vi "sub build w data.vi"(8 "error in":errorcluster, 11 "<w> data":T1) -> (0 "error out":errorcluster, 3 "<w> string":string)   [LabVIEW 2018, in "Frame Analizer.lvclass"]
uses:
  Frame Analizer.lvclass
  frame w data.ctl
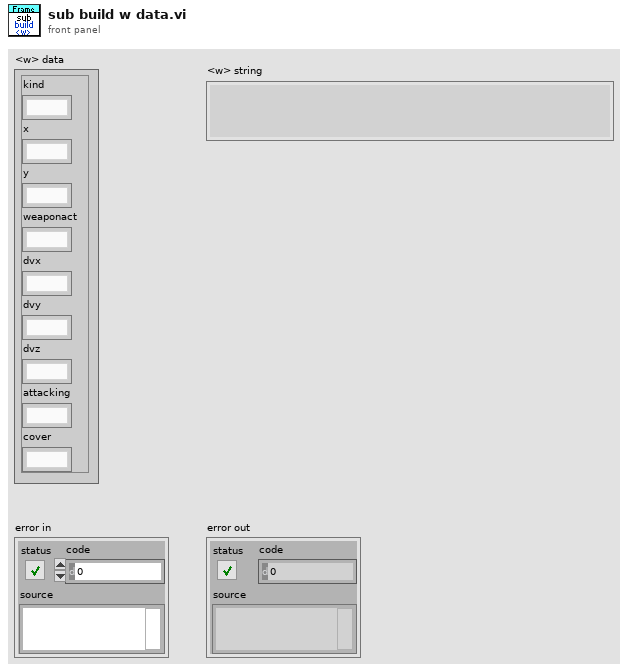
[diagram p1: front panel]
types:
  T1 = typedef "Frame Analizer.lvclass/frame w data.ctl" = cluster{"kind":string, "x":string, "y":string, "weaponact":string, "dvx":string, "dvy":string, "dvz":string, "attacking":string, "cover":string}
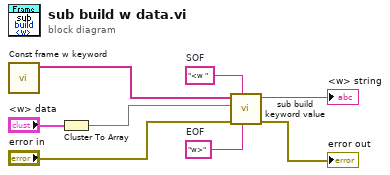
[diagram p0: block diagram]
diagram:
  w4 = "<w "  # SOF
  w2 = "w>"  # EOF
  n1 = call "Const frame w keyword.vi"() -> ("Const frame w keyword"=w1:string[])  [unwired: 11 in]
  n2 = Cluster To Array(cluster="<w> data") -> (array=w3:string[])
  n3 = call "sub build keyword value.vi"("EOF"=w2, "SOF"=w4, "error in"="error in", "value"=w3, "keyword"=w1) -> ("error out"=→"error out":errorcluster, "keyword value string"=→"<w> string":string)  [unwired: 5 in]
